vi "Get Parameter Value by Name (String).vi"(8 "Default Value":string, 9 "Parameter":string, 10 "Parameter Array in":string[](array[string])) -> (1 "Value":string, 2 "Found?":bool, 3 "Parameter Array Out":string[](array[string]))   [LabVIEW 2014]
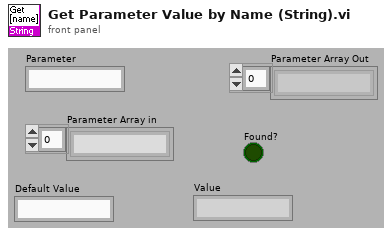
[diagram p1: front panel]
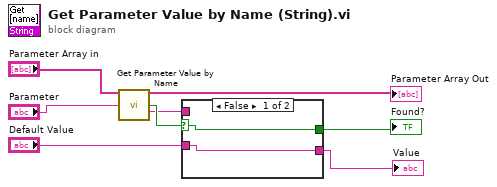
[diagram p0: block diagram]
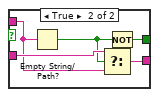
[diagram p2: hidden frame]
diagram:
  n1 = call "Get Parameter Value by Name.vi"("Parameter Array"="Parameter Array in", "Parameter Name"="Parameter") -> ("Parameter Array Out"=→"Parameter Array Out":string[], "Found?"=w5:bool, "Flattened Value"=w4:string)  [unwired: 11 in]
  n2 = case shown="False" w5 {
    selector: w5 -> [w9 _]
    tunnel: w4 -> [_ w11]
    tunnel: "Default Value" -> [w10 w14]
    tunnel: [w10 w15] -> w8
    tunnel: [w9 w13] -> w1
    frame False {
    }
    frame True {
      n3 = Empty String/Path?(string/path=w11) -> (empty?=w12:bool)
      n4 = Select(t=w14, s=w12, f=w11) -> (s? t:f=w15:string)
      n5 = Not(x=w12) -> (.not. x?=w13:bool)
    }
  }
  "Value" <- w8
  "Found?" <- w1
